vi "SLSC Get Reservation Values.vi"(8 "Error In":errorcluster, 11 "Item Ref In":T1 format="%.0x") -> (0 "Error Out":errorcluster, 1 "Reservation Access":i32(ring)=3 items=["None"=0, "Read Only"=1, "Read/Write"=3], 2 "Reservation Group":string, 3 "Item Ref Out":T1 format="%.0x")   [LabVIEW 2020, in "SLSC EDS System Explorer.lvlib"]
uses:
  System Explorer/SLSC EDS System Explorer.lvlib
  <vilib>/NI VeriStand/Custom Device API/Custom Device Item Ref.ctl
  Shared/Constants.vi
  <vilib>/NI VeriStand/Custom Device API/Get Item Property (String).vi
  <vilib>/NI VeriStand/Custom Device API/Get Item Property (I32).vi
  Shared/SLSC EDS Shared.lvlib
  <vilib>/NI VeriStand/Custom Device API/Custom Device API.lvlib
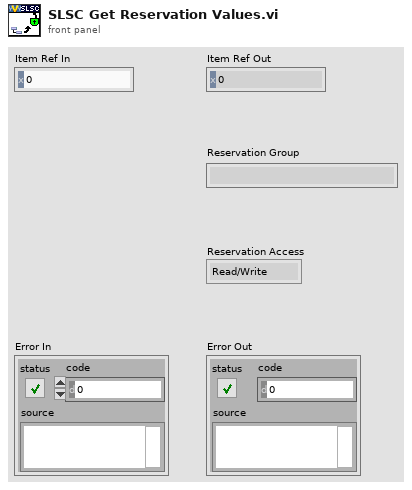
[diagram p1: front panel]
types:
  T1 = typedef "Custom Device API.lvlib/Custom Device Item Ref.ctl" = u64
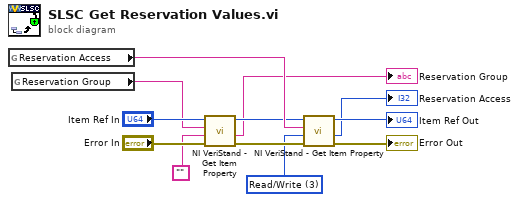
[diagram p0: block diagram]
diagram:
  w4 = 3 items=["None"=0, "Read Only"=1, "Read/Write"=3] ("Reservation Access")
  n1 = global read "Constants.vi" "Reservation Access"() -> (w8:string)
  n2 = global read "Constants.vi" "Reservation Group"() -> (w6:string)
  n3 = call-poly <vilib>:"NI VeriStand - Get Item Property.vi"("error in (no error)"="Error In", "Default Value"="", "Property Name"=w6, "Item Ref in"="Item Ref In") -> ("error out"=w11:errorcluster, "Value"=→"Reservation Group":string, "Item Ref out"=w7:T1)  [unwired: 4 in, 1 out]
  n4 = call-poly <vilib>:"NI VeriStand - Get Item Property.vi"("error in (no error)"=w11, "Default Value"=w4, "Property Name"=w8, "Item Ref in"=w7) -> ("error out"=→"Error Out":errorcluster, "Value"=→"Reservation Access":i32, "Item Ref out"=→"Item Ref Out":T1)  [unwired: 4 in, 1 out]
